vi "putForceActuatorData.vi"(8 "error in (no error)":errorcluster, 10 "TelemetryForceActuatorData":T1, 11 "Communicator in":refnum<class "Communicator.lvclass">) -> (0 "error out":errorcluster, 3 "Communicator out":refnum<class "Communicator.lvclass">)   [LabVIEW 2016, in "M1M3SupportCommunicator.lvlib" / "Communicator.lvclass"]
uses:
  Communicator.lvclass
  DataTypes/Topics/TelemetryForceActuatorData.ctl
  DataTypes/Topics/Parts/Timestamp.ctl
  DataTypes/Topics/M1M3SupportTopics.lvlib
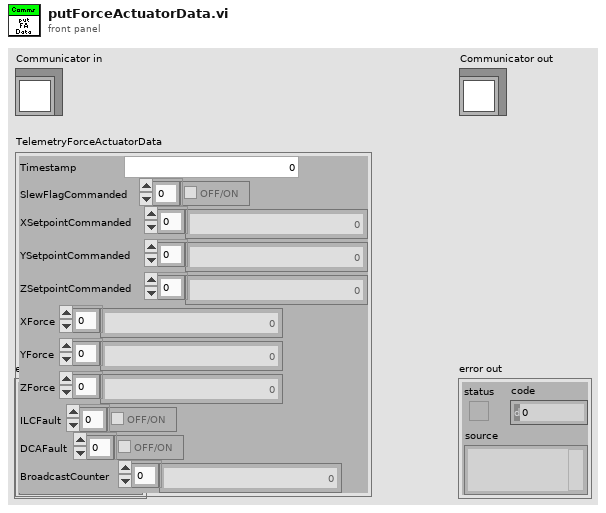
[diagram p1: front panel]
types:
  T1 = typedef "M1M3SupportTopics.lvlib/TelemetryForceActuatorData.ctl" = cluster{"Timestamp":T2, "SlewFlagCommanded":bool[], "XSetpointCommanded":dbl[], "YSetpointCommanded":dbl[], "ZSetpointCommanded":dbl[], "XForce":sgl[], "YForce":sgl[], "ZForce":sgl[], "ILCFault":bool[], "DCAFault":bool[], "BroadcastCounter":u8[]}
  T2 = typedef "M1M3SupportTopics.lvlib/Timestamp.ctl" = dbl
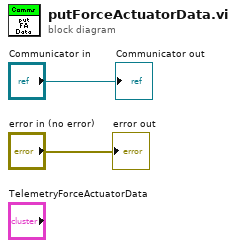
[diagram p0: block diagram]
diagram:
  "error out" <- "error in (no error)"
  "Communicator out" <- "Communicator in"
